vi "HXG2graph-scalesFGV.vi"(7 "GraphScales":T1, 8 "error in (no error)":errorcluster, 10 "Apply Scales":bool, 11 "Scales In":dbl[](array[numeric])) -> (0 "error out":errorcluster, 2 "Apply Scales":bool, 3 "Graph Scales Out":dbl[](array[numeric]))   [LabVIEW 2012]
uses:
  HXG2graphscales.ctl
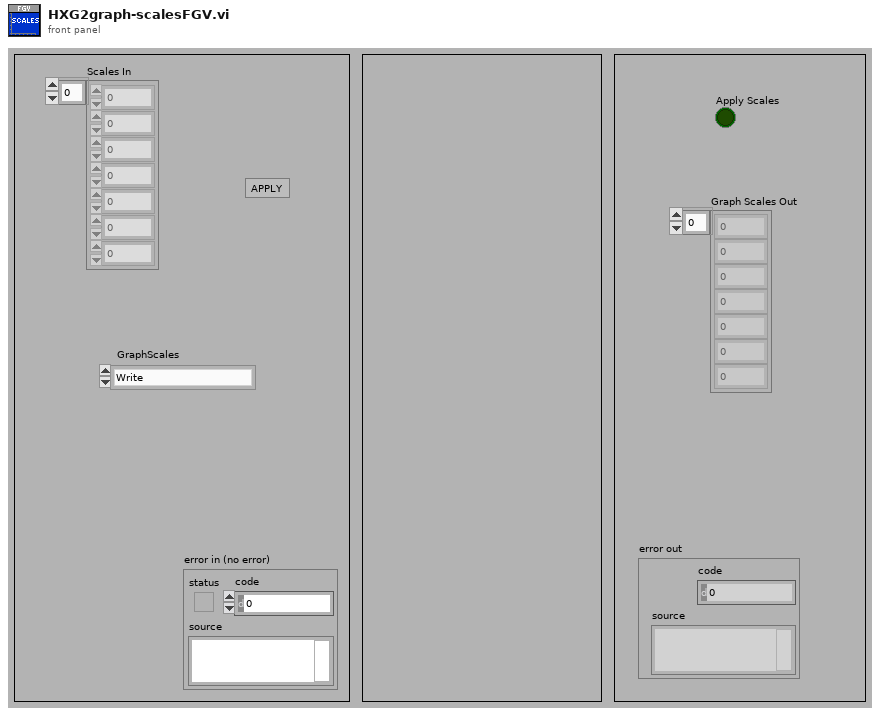
[diagram p1: front panel]
types:
  T1 = typedef "HXG2graphscales.ctl" = enum16{"Write", "Pass"}
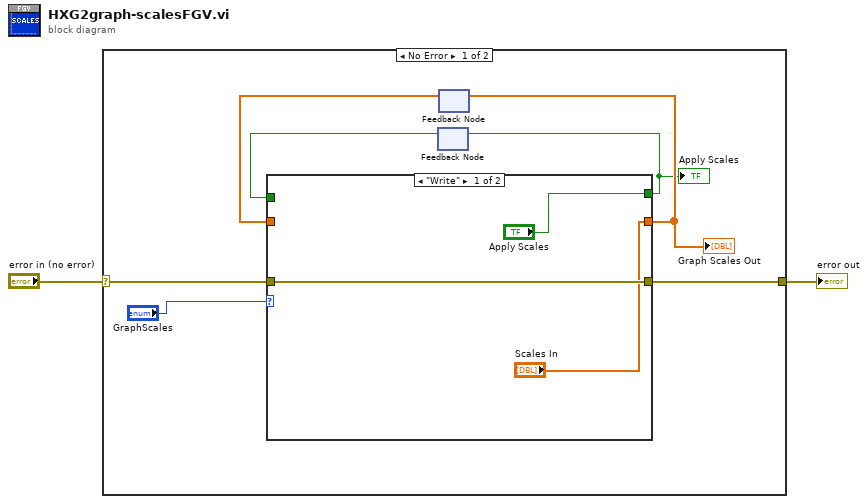
[diagram p0: block diagram]
diagram:
  n1 = case shown="No Error" "error in (no error)" {
    selector: "error in (no error)" -> [w9 w16]
    tunnel: [w8 w16] -> w1
    frame No Error {
      n2 = feedback #1() -> (w3:bool)  [unwired: 1 in]
      n3 = feedback #2() -> (w7:dbl[])  [unwired: 1 in]
      n4 = case shown="\"Write\"" "GraphScales" {
        tunnel: w9 -> [w12 w14]
        tunnel: [w12 w14] -> w8
        tunnel: ["Scales In" w15] -> w5
        tunnel: w7 -> [_ w15]
        tunnel: ["Apply Scales" w13] -> w4
        tunnel: w3 -> [_ w13]
        frame "Write" {
        }
        frame "Pass" {
        }
      }
      "Graph Scales Out" <- w5
      "Apply Scales" <- w4
      n5 = feedback-in #1(w4) -> ()
      n6 = feedback-in #2(w5) -> ()
    }
    frame Error {
    }
  }
  "error out" <- w1
